vi "Wait For Acquisition State.vi"(0 "fpga interface in":refnum<k20>, 5 "global acq state":T1[](array[typedef]), 9 "timeout (s)":dbl=1.0, 11 "error in (no error)":errorcluster) -> (4 "fpga interface out":refnum<k20>, 15 "error out":errorcluster)   [LabVIEW 2023, in "GettingStarted_Acq_148X_Host.lvlib"]
uses:
  GettingStarted_Acq_148X_Host.lvlib
  <instrlib>/FlexRIO/CSI-2/v2/FPGA/Types/Global Acquisition Engine State.ctl
  Types/148x_Acq_FPGA_Reference.ctl
  <vilib>/rvi/errors/niLvFpgaAdjustHostInterfaceError.vi
  <vilib>/rvi/interface/nirviReadWriteControl/nirviReadWriteControl.xnode
  NiFpgaLv.dll
  <vilib>/rvi/interface/Simulation/niFpgaSimulationCallBeginRW.vi
  <instrlib>/FlexRIO/CSI-2/v2/FPGA/NI CSI-2 API FPGA v2.lvlib
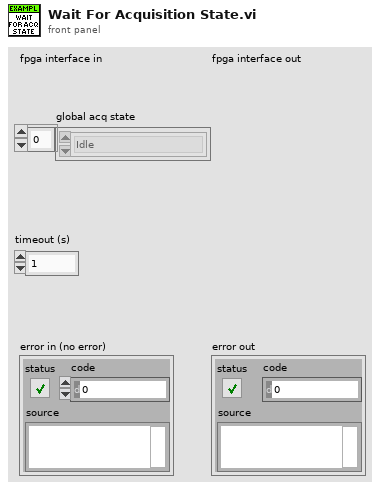
[diagram p1: front panel]
types:
  T1 = typedef "NI CSI-2 API FPGA v2.lvlib/Global Acquisition Engine State.ctl" = enum8{"Idle", "Ready For Start Trigger", "Acquire", "Error"}
  T2 = typedef "GettingStarted_Acq_148X_Host.lvlib/148x_Acq_FPGA_Reference.ctl" = refnum<k20>
  T3 = enum8{"Idle", "Ready For Start Trigger", "Acquire", "Error"}
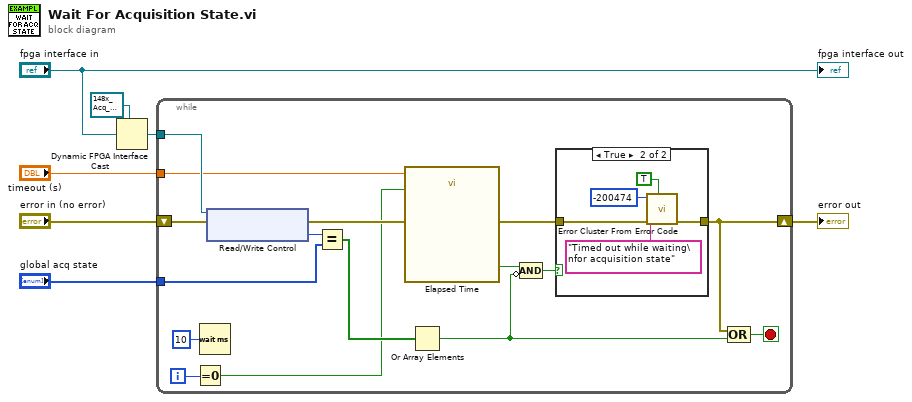
[diagram p0: block diagram]
diagram:
  n1 = Dynamic FPGA Interface Cast(Session In=T2 refnum ("FPGA VI Reference Out"), Type="fpga interface in") -> (Session Out=w3:T2)
  n2 = while {
    tunnel: w3 -> [w23]
    tunnel: "global acq state" -> [w21]
    shift-right: [w15] -> w7
    shift-left: "error in (no error)" -> [w19]
    tunnel: "timeout (s)" -> [w17]
    i -> [w11]
    stop <- w20 stop-if-true
    n3 = Equal To 0?(x=w11) -> (x = 0?=w10:bool)
    n4 = Wait (ms)(milliseconds to wait=u32 10) -> ()  [unwired: 1 out]
    n5 = xnode "Read/Write Control"("FPGA VI Reference In"=w23, "error in"=w19) -> ("error out"=w18:errorcluster, "global acq state"=w22:T3)  [unwired: 1 out]
    n6 = Equal?(x=w22, y=w21) -> (x = y?=w12:bool[])
    n7 = call "Elapsed Time"("Time Target (s)"=w17, "Reset"=w10, "error in (no error)"=w18) -> ("Time has Elapsed"=w14:bool, "error out"=w16:errorcluster)  [unwired: 9 in, 6 out]
    n8 = Or Array Elements(Boolean array=w12) -> (logical OR=w8:bool)
    n9 = Compound Arithmetic op=AND(w14, invert w8) -> (w13:bool)
    n10 = case shown="True" w13 {
      tunnel: w16 -> [w24 w28]
      tunnel: [w24 w27] -> w15
      frame False {
      }
      frame True {
        n11 = call <vilib>:"Error Cluster From Error Code.vi"("show call chain? (False)"=TRUE, "error in (no error)"=w28, "error message (\"\")"="Timed out while waiting\nfor acquisition state" ("error message (\"\")"), "error code (0)"=-200474) -> ("error out"=w27:errorcluster)  [unwired: 5 in]
      }
    }
    n12 = Compound Arithmetic op=OR(w15, w8) -> (w20:bool)
  }
  "error out" <- w7
  "fpga interface out" <- "fpga interface in"
